vi "Slave_ID.vi"(6 "New ID":u8 format="%07b", 7 "I2C Channel":u8, 8 "error in (no error)":errorcluster, 10 "ID  Action":enum16{"Read ID", "Write ID"}(ring), 11 "LINX Resource In":T1) -> (0 "error out":errorcluster, 2 "Slave ID Out":u8 format="%08b", 3 "LINX Resource Out":T1)   [LabVIEW 2014, in "LMH-LINX.lvlib" / "ITG3200.lvlib"]
uses:
  <vilib>/MakerHub/LINX/Public/Sensors/Gyroscopes/ITG3200/ITG3200.lvlib
  <vilib>/MakerHub/LINX/Private/Type Defs/LINX Ref.ctl
  <vilib>/MakerHub/LINX/Private/Type Defs/Platform.ctl
  <vilib>/MakerHub/LINX/Private/Type Defs/Interface.ctl
  <vilib>/MakerHub/LINX/Private/Device/Type Defs/LINX Device Config.ctl
  <vilib>/MakerHub/LINX/Private/Device/Type Defs/TCP Config.ctl
  <vilib>/MakerHub/LINX/Private/Device/Type Defs/Channels.ctl
  <vilib>/MakerHub/LINX/Private/Local IO/LinxI2cWrite.vi
  <vilib>/MakerHub/LINX/Public/Utilities/Check Channel.vi
  <vilib>/MakerHub/LINX/Private/Utilties/Generate Error.vi
  <vilib>/MakerHub/LINX/LMH-LINX.lvlib
  <vilib>/MakerHub/LINX/Private/Device/Device.lvlib
panel:
  # "OUTPUTS"
  # "INPUTS"
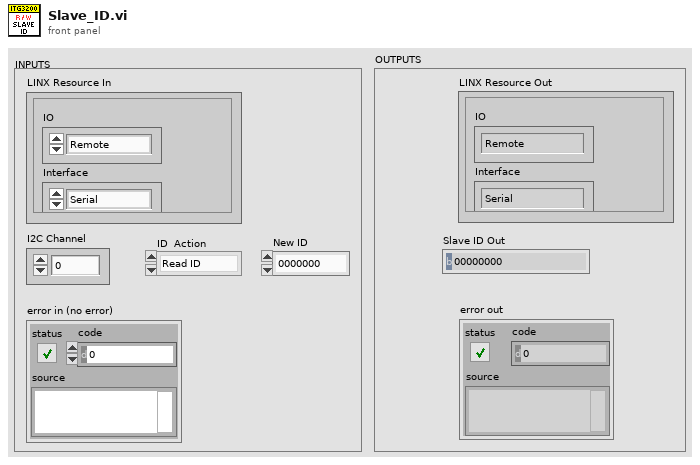
[diagram p1: front panel]
types:
  T1 = typedef "LMH-LINX.lvlib/LINX Ref.ctl" = cluster{"IO":T2, "Interface":T3, "LINX Device Config":T4}
  T2 = typedef "LMH-LINX.lvlib/Platform.ctl" = enum16{"Remote", "Local"}
  T3 = typedef "LMH-LINX.lvlib/Interface.ctl" = enum16{"Serial", "TCP"}
  T4 = typedef "LMH-LINX.lvlib/Device.lvlib/LINX Device Config.ctl" = cluster{"Interface":T3, "COM Port":refnum<visa-resource-name>, "TCP Configuration":T5, "Device Family":u8, "Device ID":u8, "Device Name":string, "TCP Ref":refnum<k5>, "Channels":T6}
  T5 = typedef "LMH-LINX.lvlib/Device.lvlib/TCP Config.ctl" = cluster{"IP Address":string, "Port":u16}
  T6 = typedef "LMH-LINX.lvlib/Channels.ctl" = cluster{"DI":u8[], "DO":u8[], "AI":u8[], "AO":u8[], "PWM":u8[], "QE":u8[], "UART":u8[], "I2C 2":u8[], "SPI":u8[], "CAN":u8[], "Servo":u8[], "AI Ref (V)":dbl, "AI Resolution (Bits)":u8, "AO Ref (V)":dbl, "AO Resolution (Bits)":u8}
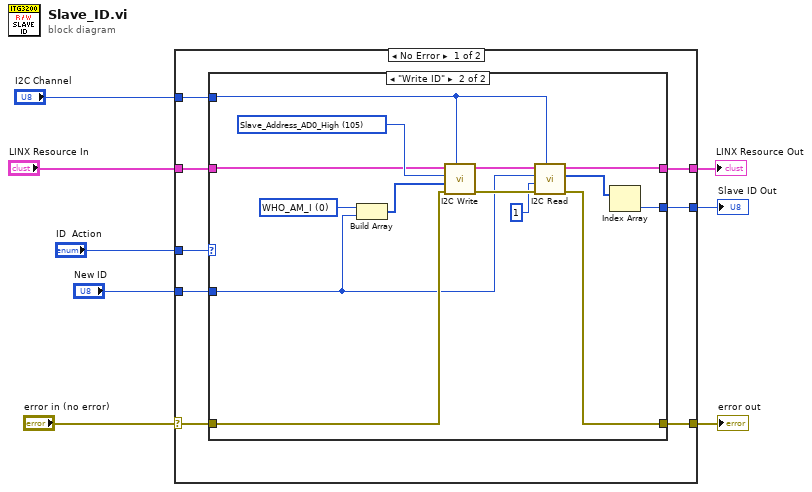
[diagram p0: block diagram]
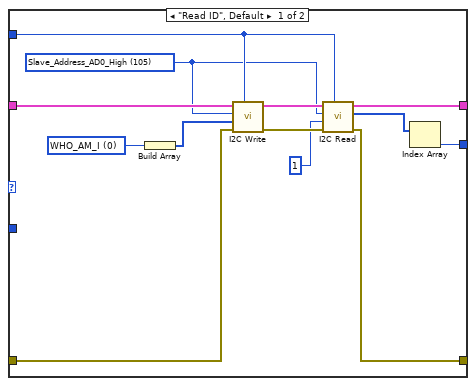
[diagram p2: hidden frame]
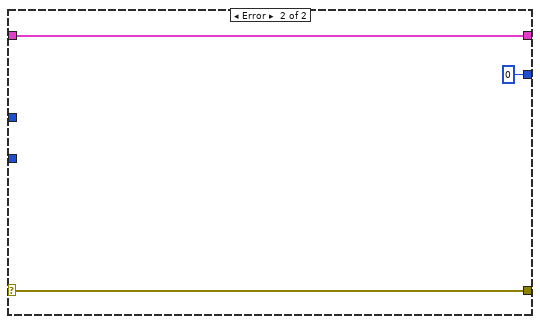
[diagram p3: hidden frame]
diagram:
  n1 = case shown="No Error" "error in (no error)" {
    selector: "error in (no error)" -> [w15 w46]
    tunnel: [w14 w46] -> w7
    tunnel: "LINX Resource In" -> [w16 w45]
    tunnel: "I2C Channel" -> [w12 _]
    tunnel: [w13 w45] -> w4
    tunnel: [w11 u8 0 ("element")] -> w3
    tunnel: "ID  Action" -> [w10 _]
    tunnel: "New ID" -> [w9 _]
    frame No Error {
      n2 = case shown="\"Write ID\"" w10 {
        tunnel: w16 -> [w29 w35]
        tunnel: w15 -> [w28 w32]
        tunnel: [w23 w31] -> w14
        tunnel: [w22 w34] -> w13
        tunnel: w12 -> [w21 w36]
        tunnel: [w17 w33] -> w11
        tunnel: w9 -> [_ w30]
        frame "Read ID", Default {
          w27 = u8 0 items=["WHO_AM_I"=0, "SMPLRT_DIV"=21, "DLPF_FS"=22, "INT_CFG"=23, "INT_STATUS"=26, "TEMP_OUT_H"=27, "TEMP_OUT_L"=28, "GYRO_XOUT_H"=29, "GYRO_XOUT_L"=30, "GYRO_YOUT_H"=31, "GYRO_YOUT_L"=32, "GYRO_ZOUT_H"=33, "GYRO_ZOUT_L"=34, "PWR_MGM"=62] ("Register Map")
          w20 = u8 105 items=["Slave_Address_AD0_Low"=104, "Slave_Address_AD0_High"=105] ("Slave Addresses")
          n3 = Build Array(w27) -> (w26:u8[])
          n4 = call <vilib>:"I2C Write.vi"("I2C Channel"=w21, "Error In"=w28, "Data"=w26, "I2C Slave Address (0)"=w20, "LINX Resource"=w29) -> ("Error Out"=w24:errorcluster, "LINX Resource"=w25:T1)  [unwired: 5 in]
          n5 = call <vilib>:"I2C Read.vi"("I2C Channel"=w21, "Error In"=w24, "Bytes To Read"=u8 1, "I2C Slave Address (0)"=w20, "LINX Resource"=w25) -> ("Error Out"=w23:errorcluster, "Data"=w18:u8[], "LINX Resource"=w22:T1)  [unwired: 4 in]
          n6 = Index Array(array=w18) -> (element=w17:u8)  [unwired: 1 in]
        }
        frame "Write ID" {
          w43 = u8 0 items=["WHO_AM_I"=0, "SMPLRT_DIV"=21, "DLPF_FS"=22, "INT_CFG"=23, "INT_STATUS"=26, "TEMP_OUT_H"=27, "TEMP_OUT_L"=28, "GYRO_XOUT_H"=29, "GYRO_XOUT_L"=30, "GYRO_YOUT_H"=31, "GYRO_YOUT_L"=32, "GYRO_ZOUT_H"=33, "GYRO_ZOUT_L"=34, "PWR_MGM"=62] ("Register Map")
          w39 = u8 105 items=["Slave_Address_AD0_Low"=104, "Slave_Address_AD0_High"=105] ("Slave Addresses")
          n7 = Build Array(w43, w30) -> (w42:u8[])
          n8 = call <vilib>:"I2C Write.vi"("I2C Channel"=w36, "Error In"=w32, "Data"=w42, "I2C Slave Address (0)"=w39, "LINX Resource"=w35) -> ("Error Out"=w40:errorcluster, "LINX Resource"=w41:T1)  [unwired: 5 in]
          n9 = call <vilib>:"I2C Read.vi"("I2C Channel"=w36, "Error In"=w40, "Bytes To Read"=u8 1, "I2C Slave Address (0)"=w30, "LINX Resource"=w41) -> ("Error Out"=w31:errorcluster, "Data"=w37:u8[], "LINX Resource"=w34:T1)  [unwired: 4 in]
          n10 = Index Array(array=w37) -> (element=w33:u8)  [unwired: 1 in]
        }
      }
    }
    frame Error {
    }
  }
  "error out" <- w7
  "LINX Resource Out" <- w4
  "Slave ID Out" <- w3
